vi "采集参数设置 - 副本.vi"() -> ()   [LabVIEW 2020]
panel:
  in  "物理量8下限":sgl format="%#.4g"
  in  "物理量8上限":sgl format="%#.4g"
  in  "物理量7下限":sgl format="%#.4g"
  in  "物理量7上限":sgl format="%#.4g"
  in  "物理量6下限":sgl format="%#.4g"
  in  "物理量6上限":sgl format="%#.4g"
  in  "物理量5下限":sgl format="%#.4g"
  in  "物理量5上限":sgl format="%#.4g"
  in  "物理量4下限":sgl format="%#.4g"
  in  "物理量4上限":sgl format="%#.4g"
  in  "物理量3下限":sgl format="%#.4g"
  in  "物理量3上限":sgl format="%#.4g"
  in  "物理量2下限":sgl format="%#.4g"
  in  "物理量2上限":sgl format="%#.4g"
  in  "物理量1下限":sgl format="%#.4g"
  in  "物理量1上限":sgl format="%#.4g"
  in  "网络服务标尺":u16(ring) items=["计数通量", "电压通量", "电流通量", "棒位", "温度", "P2参数", "硼浓度"]
  in  "端口：":u16=502
  in  "DCS服务器IP地址/主机名：":string="192.168.1.2"
  in  "反应性仪IP地址/主机名：":string="192.168.1.15"
  in  "电压下限8":i32(slide) scale=-10.0..1.0
  in  "电压范围8":i32(slide) scale=1.0..10.0
  in  "电压下限7":i32(slide) scale=-10.0..1.0
  in  "电压范围7":i32(slide) scale=1.0..10.0
  in  "电压下限6":i32(slide) scale=-10.0..1.0
  in  "电压范围6":i32(slide) scale=1.0..10.0
  in  "电压下限5":i32(slide) scale=-10.0..1.0
  in  "电压范围5":i32(slide) scale=1.0..10.0
  in  "电压下限4":i32(slide) scale=-10.0..1.0
  in  "电压范围4":i32(slide) scale=1.0..10.0
  in  "电压下限3":i32(slide) scale=-10.0..1.0
  in  "电压范围3":i32(slide) scale=1.0..10.0
  in  "电压下限2":i32(slide) scale=-10.0..1.0
  in  "电压范围2":i32(slide) scale=1.0..10.0
  in  "电压下限1":i32(slide) scale=-10.0..1.0
  in  "电压范围1":i32(slide) scale=1.0..10.0
  in  "电压标尺8":u16(ring) items=["计数通量LOG", "电压通量", "电流通量LOG", "棒位", "温度", "P2参数", "硼浓度"]
  in  "电压标尺7":u16(ring) items=["计数通量LOG", "电压通量", "电流通量LOG", "棒位", "温度", "P2参数", "硼浓度"]
  in  "电压标尺6":u16(ring) items=["计数通量LOG", "电压通量", "电流通量LOG", "棒位", "温度", "P2参数", "硼浓度"]
  in  "电压标尺5":u16(ring) items=["计数通量LOG", "电压通量", "电流通量LOG", "棒位", "温度", "P2参数", "硼浓度"]
  in  "电压标尺4":u16(ring) items=["计数通量LOG", "电压通量", "电流通量LOG", "棒位", "温度", "P2参数", "硼浓度"]
  in  "电压标尺3":u16(ring) items=["计数通量LOG", "电压通量", "电流通量LOG", "棒位", "温度", "P2参数", "硼浓度"]
  in  "电压标尺2":u16(ring) items=["计数通量LOG", "电压通量", "电流通量LOG", "棒位", "温度", "P2参数", "硼浓度"]
  in  "电压标尺1":u16(ring) items=["计数通量LOG", "电压通量", "电流通量LOG", "棒位", "温度", "P2参数", "硼浓度"]
  in  "电流输入名称2":string
  in  "电流输入名称1":string
  in  "电压输入名称8":string
  in  "电压输入名称7":string
  in  "电压输入名称6":string
  in  "电压输入名称5":string
  in  "电压输入名称4":string
  in  "电压输入名称3":string
  in  "电压输入名称2":string
  in  "电压输入名称1":string
  in  "脉冲输入名称3":string
  in  "脉冲输入名称2":string
  in  "脉冲输入名称1":string
  in  "DCS服务器连接：":bool
  in  "反应性仪连接：":bool
  in  "电流输入2":bool
  in  "电流输入1":bool
  in  "电压输入8":bool
  in  "电压输入7":bool
  in  "电压输入6":bool
  in  "电压输入5":bool
  in  "电压输入4":bool
  in  "恢复":bool caption="Cancel Button"
  out "脉冲3":bool
  out "脉冲2":bool
  in  "电压输入3":bool
  in  "电压输入2":bool
  in  "电压输入1":bool
  out "脉冲1":bool
  in  "脉冲计数通道2":bool
  in  "脉冲计数通道3":bool
  in  "脉冲计数通道1":bool
  in  "取消修改":bool caption="Cancel Button"
  in  "保存修改":bool
  in  "采集时间间隔(s)：":sgl(knob)=0.5 min=0.5 max=2 step=0.5 scale=0.5..2.0 scale format="%#.1f"
  # "仪器硬件通讯设置"
  # "电压输入通道"
  # "电流输入通道"
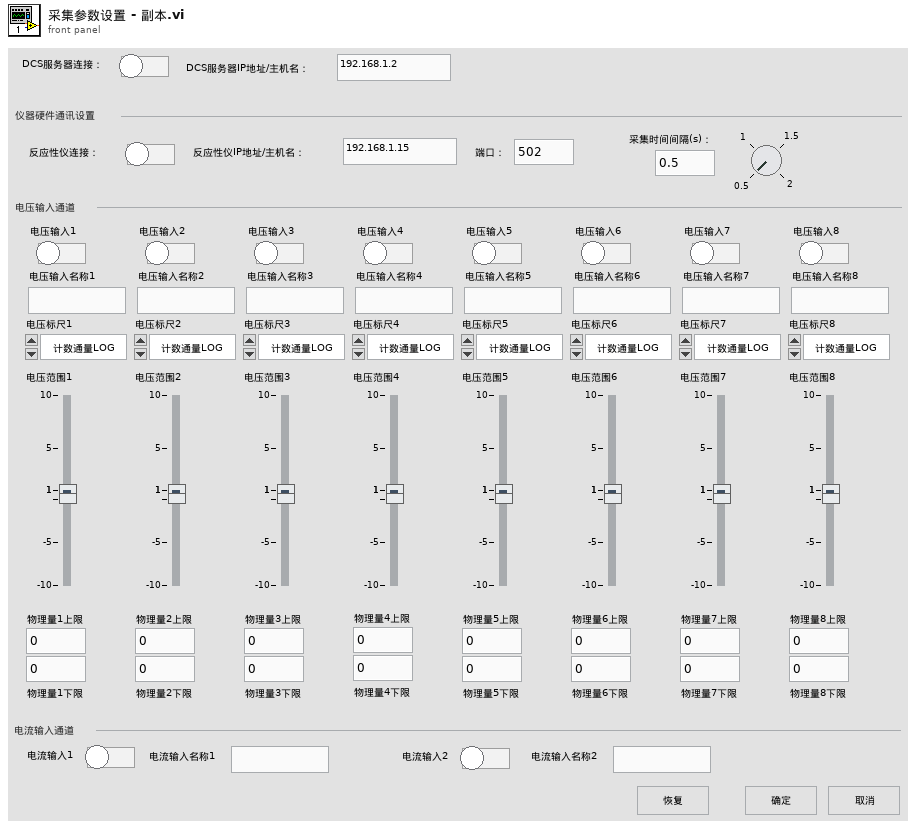
[diagram p1: front panel]
types:
  T1 = enum16{"open", "replace", "create", "open or create", "replace or create", "replace or create with confirmation"}
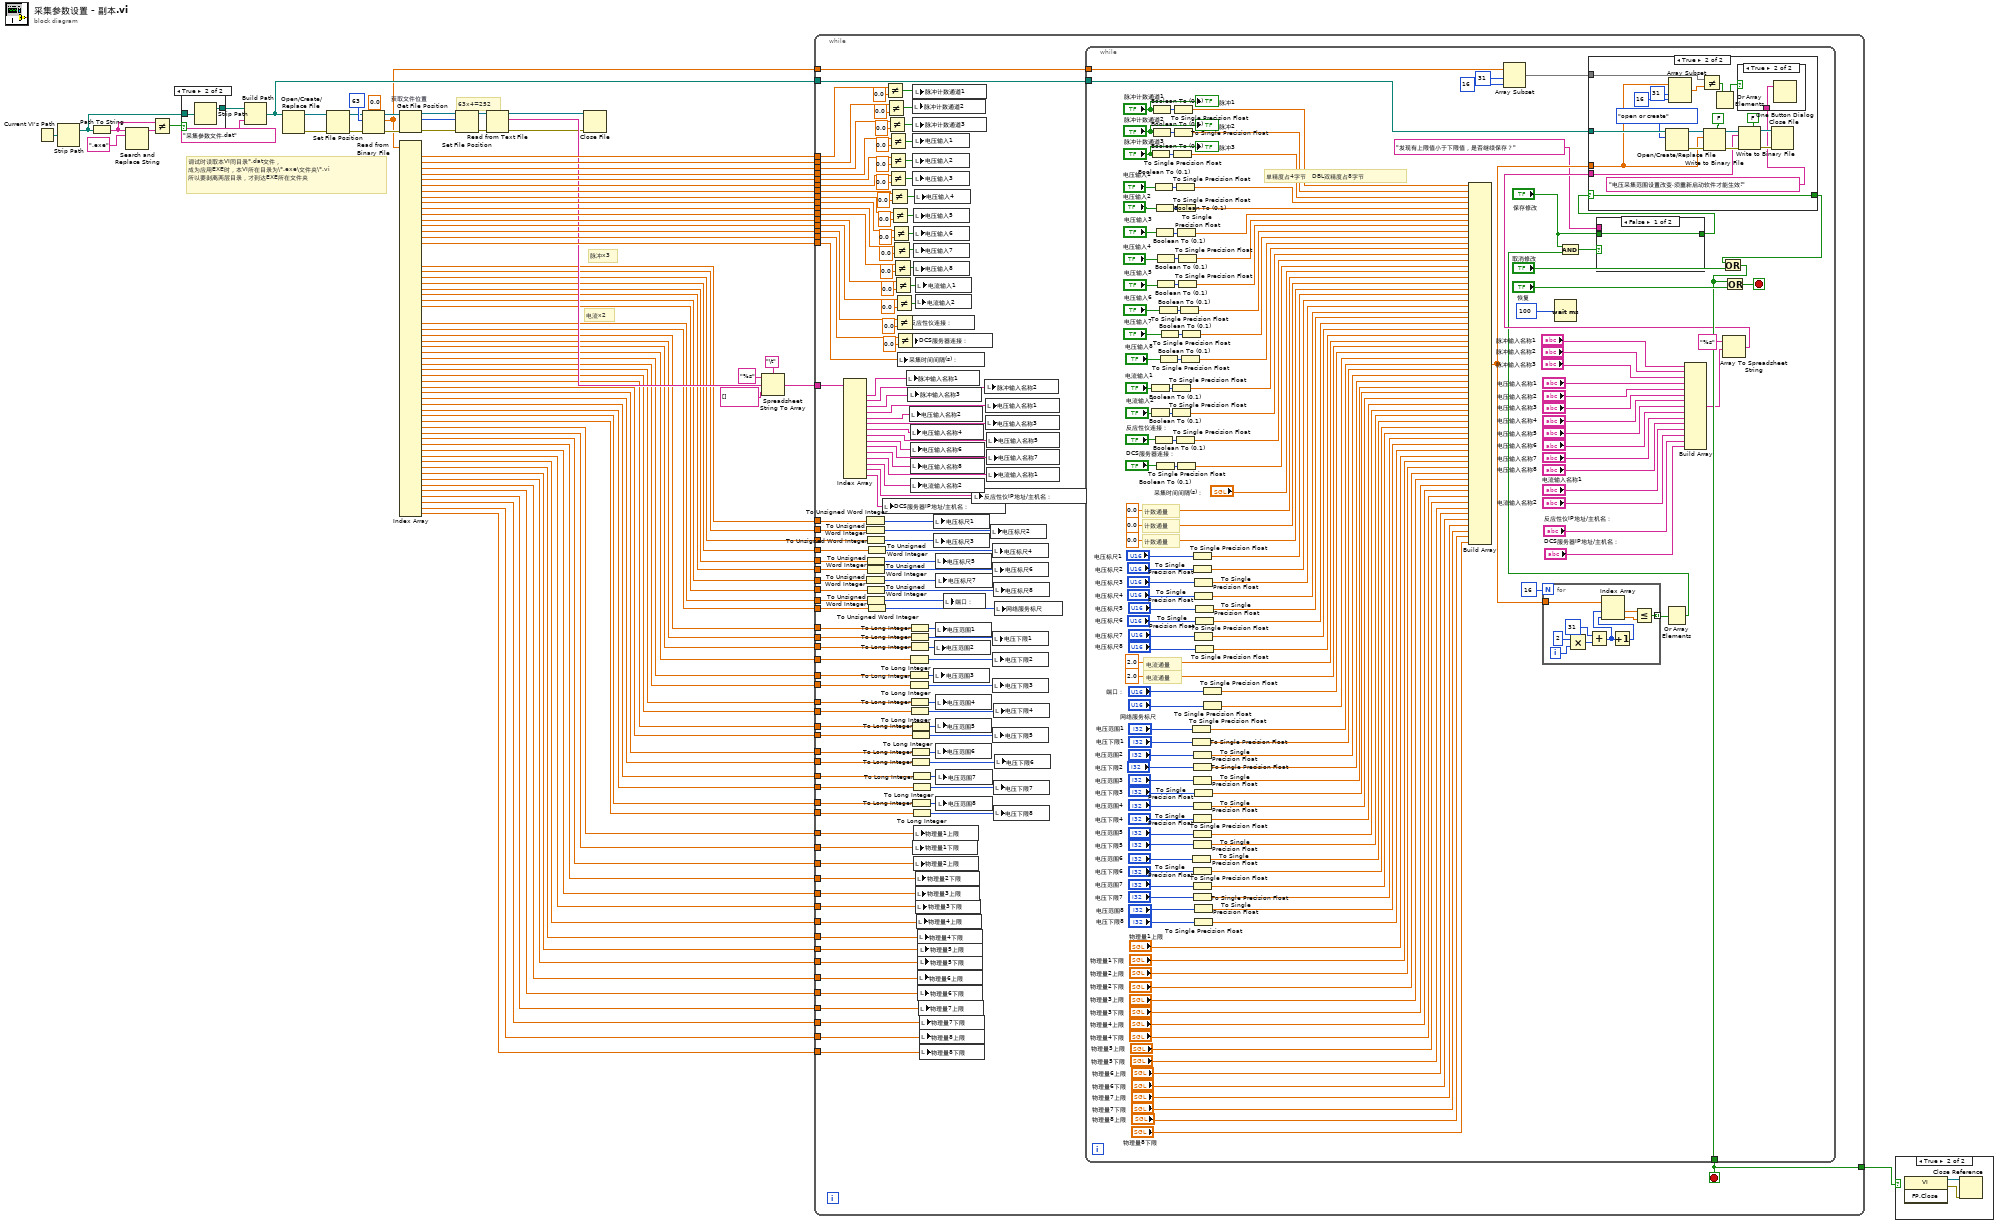
[diagram p0: block diagram]
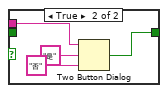
[diagram p4: hidden frame]
diagram:
  # "调试时读取本VI同目录*.dat文件，\n成为应用EXE时，本VI所在目录为\\*.exe\\文件夹\\*.vi\n所以要剥离两层目录，才到达EXE所在文件夹"
  # "63x4=252"
  # "电流x2"
  # "脉冲x3"
  n1 = Current VI's Path() -> (path=w29:path)
  n2 = Strip Path(path=w29) -> (stripped path=w24:path)  [unwired: 1 out]
  n3 = Path To String(path=w24) -> (string=w26:string)
  n4 = Search and Replace String(input string=w26, search string=".exe" ("搜索字符串")) -> (result string=w27:string)  [unwired: 6 in, 3 out]
  n5 = Not Equal?(x=w26, y=w27) -> (x != y?=w25:bool)
  n6 = case shown="True" w25 {
    tunnel: w24 -> [w90 w92]
    tunnel: [w90 w91] -> w23
    frame False {
    }
    frame True {
      n7 = Strip Path(path=w92) -> (stripped path=w91:path)  [unwired: 1 out]
    }
  }
  n8 = Build Path(base path=w23, name or relative path="采集参数文件.dat") -> (appended path=w84:path)
  n9 = Open/Create/Replace File(file path (use dialog)=w84) -> (refnum out=w67:refnum<file>, error out=w66:errorcluster)  [unwired: 5 in, 1 out]
  n10 = Set File Position(refnum=w67, error in=w66) -> (refnum out=w65:refnum<file>, error out=w64:errorcluster)  [unwired: 2 in]
  n11 = Read from Binary File(5:sgl 0.0 ("byte stream type"), 8:w64, 10:63 ("count"), 11:w65) -> (0:w82:errorcluster, 2:w4:sgl[], 3:w83:refnum<file>)  [unwired: 2 in, 1 out]
  n12 = Get File Position "获取文件位置"(4:w82, 7:w83) -> (0:w86:errorcluster, 2:w52:i64, 3:w87:refnum<file>)
  n13 = Index Array(array=w4) -> (element #1=w81:sgl, element #2=w80:sgl, element #3=w79:sgl, element #4=w78:sgl, element #5=w77:sgl, element #6=w76:sgl, element #7=w75:sgl, element #8=w74:sgl, element #9=w73:sgl, element #10=w72:sgl, element #11=w71:sgl, element #12=w70:sgl, element #13=w69:sgl, element #14=w68:sgl, element #15=w63:sgl, element #16=w62:sgl, element #20=w51:sgl, element #21=w50:sgl, element #22=w49:sgl, element #23=w48:sgl, element #24=w47:sgl, element #25=w46:sgl, element #26=w45:sgl, element #27=w44:sgl, element #30=w2:sgl, element #31=w3:sgl, element #32=w43:sgl, element #33=w42:sgl, element #34=w41:sgl, element #35=w40:sgl, element #36=w21:sgl, element #37=w22:sgl, element #38=w39:sgl, element #39=w38:sgl, element #40=w37:sgl, element #41=w36:sgl, element #42=w35:sgl, element #43=w34:sgl, element #44=w33:sgl, element #45=w32:sgl, element #46=w31:sgl, element #47=w30:sgl, element #48=w20:sgl, element #49=w19:sgl, element #50=w18:sgl, element #51=w17:sgl, element #52=w16:sgl, element #53=w15:sgl, element #54=w14:sgl, element #55=w13:sgl, element #56=w12:sgl, element #57=w11:sgl, element #58=w10:sgl, element #59=w9:sgl, element #60=w8:sgl, element #61=w7:sgl, element #62=w6:sgl, element #63=w5:sgl)  [unwired: 63 in, 5 out]
  n14 = Set File Position(offset (in bytes) (0)=w52, refnum=w87, error in=w86) -> (refnum out=w59:refnum<file>, error out=w58:errorcluster)  [unwired: 1 in]
  n15 = Read from Text File(file (use dialog)=w59, error in=w58) -> (refnum out=w54:refnum<file>, text=w57:string, error out=w55:errorcluster)  [unwired: 1 in, 2 out]
  n16 = Close File(refnum=w54, error in=w55) -> ()  [unwired: 2 out]
  n17 = Spreadsheet String To Array(delimiter (Tab)="\t", format string="%s", spreadsheet string=w57, array type (2D Dbl)=string[] [] ("添加的数组")) -> (array=w53:string[])
  n18 = while {
    tunnel: w81 -> [w224]
    tunnel: w80 -> [w218]
    tunnel: w79 -> [w217]
    tunnel: w78 -> [w216]
    tunnel: w77 -> [w210]
    tunnel: w76 -> [w208]
    tunnel: w75 -> [w196]
    tunnel: w74 -> [w195]
    tunnel: w73 -> [w194]
    tunnel: w72 -> [w193]
    tunnel: w71 -> [w192]
    tunnel: w70 -> [w183]
    tunnel: w84 -> [w225]
    tunnel: w69 -> [w182]
    tunnel: w68 -> [w181]
    tunnel: w63 -> [w180]
    tunnel: w62 -> [w179]
    tunnel: w53 -> [w178]
    tunnel: w51 -> [w156]
    tunnel: w50 -> [w155]
    tunnel: w49 -> [w154]
    tunnel: w48 -> [w153]
    tunnel: w47 -> [w152]
    tunnel: w46 -> [w151]
    tunnel: w45 -> [w150]
    tunnel: w44 -> [w149]
    tunnel: w2 -> [w114]
    tunnel: w3 -> [w113]
    tunnel: w41 -> [w132]
    tunnel: w40 -> [w131]
    tunnel: w21 -> [w130]
    tunnel: w22 -> [w129]
    tunnel: w39 -> [w128]
    tunnel: w38 -> [w127]
    tunnel: w37 -> [w126]
    tunnel: w36 -> [w125]
    tunnel: w35 -> [w124]
    tunnel: w34 -> [w123]
    tunnel: w33 -> [w122]
    tunnel: w32 -> [w121]
    tunnel: w31 -> [w120]
    tunnel: w30 -> [w119]
    tunnel: w43 -> [w112]
    tunnel: w42 -> [w111]
    tunnel: w20 -> [w110]
    tunnel: w19 -> [w109]
    tunnel: w18 -> [w108]
    tunnel: w17 -> [w107]
    tunnel: w16 -> [w106]
    tunnel: w15 -> [w105]
    tunnel: w14 -> [w104]
    tunnel: w13 -> [w103]
    tunnel: w12 -> [w102]
    tunnel: w11 -> [w101]
    tunnel: w10 -> [w100]
    tunnel: w9 -> [w99]
    tunnel: w8 -> [w98]
    tunnel: w7 -> [w97]
    tunnel: w6 -> [w96]
    tunnel: w5 -> [w95]
    tunnel: w4 -> [w94]
    tunnel: [w93] -> w1
    stop <- w93 stop-if-true
    n19 = Index Array(array=w178) -> (element #1=w177:string, element #2=w176:string, element #3=w175:string, element #4=w174:string, element #5=w173:string, element #6=w172:string, element #7=w171:string, element #8=w170:string, element #9=w169:string, element #10=w168:string, element #11=w167:string, element #12=w165:string, element #13=w166:string, element #14=w118:string, element #15=w117:string)  [unwired: 15 in]
    n20 = To Unsigned Word Integer(number=w156) -> (unsigned 16bit integer=w164:u16)
    n21 = To Unsigned Word Integer(number=w155) -> (unsigned 16bit integer=w162:u16)
    n22 = To Unsigned Word Integer(number=w150) -> (unsigned 16bit integer=w158:u16)
    n23 = To Unsigned Word Integer(number=w154) -> (unsigned 16bit integer=w163:u16)
    n24 = To Unsigned Word Integer(number=w152) -> (unsigned 16bit integer=w160:u16)
    n25 = To Unsigned Word Integer(number=w151) -> (unsigned 16bit integer=w159:u16)
    n26 = To Unsigned Word Integer(number=w149) -> (unsigned 16bit integer=w157:u16)
    n27 = To Unsigned Word Integer(number=w114) -> (unsigned 16bit integer=w116:u16)
    n28 = To Unsigned Word Integer(number=w153) -> (unsigned 16bit integer=w161:u16)
    n29 = To Unsigned Word Integer(number=w113) -> (unsigned 16bit integer=w115:u16)
    n30 = local write "DCS服务器IP地址/主机名："(w117) -> ()
    n31 = Not Equal?(x=w224, y=sgl 0.0) -> (x != y?=w222:bool)
    n32 = Not Equal?(x=w218, y=sgl 0.0) -> (x != y?=w215:bool)
    n33 = Not Equal?(x=w217, y=sgl 0.0) -> (x != y?=w214:bool)
    n34 = Not Equal?(x=w216, y=sgl 0.0) -> (x != y?=w213:bool)
    n35 = Not Equal?(x=w210, y=sgl 0.0) -> (x != y?=w211:bool)
    n36 = Not Equal?(x=w208, y=sgl 0.0) -> (x != y?=w207:bool)
    n37 = Not Equal?(x=w196, y=sgl 0.0) -> (x != y?=w201:bool)
    n38 = Not Equal?(x=w195, y=sgl 0.0) -> (x != y?=w200:bool)
    n39 = Not Equal?(x=w194, y=sgl 0.0) -> (x != y?=w199:bool)
    n40 = Not Equal?(x=w193, y=sgl 0.0) -> (x != y?=w198:bool)
    n41 = Not Equal?(x=w192, y=sgl 0.0) -> (x != y?=w197:bool)
    n42 = Not Equal?(x=w183, y=sgl 0.0) -> (x != y?=w185:bool)
    n43 = Not Equal?(x=w182, y=sgl 0.0) -> (x != y?=w184:bool)
    n44 = Not Equal?(x=w181, y=sgl 0.0) -> (x != y?=w189:bool)
    n45 = Not Equal?(x=w180, y=sgl 0.0) -> (x != y?=w188:bool)
    n46 = local write "采集时间间隔(s)："(w179) -> ()
    n47 = local write "反应性仪连接："(w189) -> ()
    n48 = local write "脉冲输入名称1"(w177) -> ()
    n49 = local write "DCS服务器连接："(w188) -> ()
    n50 = local write "脉冲输入名称3"(w175) -> ()
    n51 = To Long Integer(number=w131) -> (32bit integer=w139:i32)
    n52 = To Long Integer(number=w130) -> (32bit integer=w146:i32)
    n53 = To Long Integer(number=w129) -> (32bit integer=w138:i32)
    n54 = To Long Integer(number=w112) -> (32bit integer=w148:i32)
    n55 = To Long Integer(number=w111) -> (32bit integer=w140:i32)
    n56 = To Long Integer(number=w132) -> (32bit integer=w147:i32)
    n57 = To Long Integer(number=w128) -> (32bit integer=w145:i32)
    n58 = To Long Integer(number=w127) -> (32bit integer=w137:i32)
    n59 = local write "电压输入名称2"(w173) -> ()
    n60 = To Long Integer(number=w126) -> (32bit integer=w144:i32)
    n61 = To Long Integer(number=w125) -> (32bit integer=w136:i32)
    n62 = To Long Integer(number=w124) -> (32bit integer=w143:i32)
    n63 = To Long Integer(number=w123) -> (32bit integer=w135:i32)
    n64 = local write "电压输入名称4"(w171) -> ()
    n65 = To Long Integer(number=w120) -> (32bit integer=w141:i32)
    n66 = local write "电压输入名称6"(w169) -> ()
    n67 = local write "电压输入名称8"(w167) -> ()
    n68 = local write "电流输入名称2"(w166) -> ()
    n69 = To Long Integer(number=w122) -> (32bit integer=w142:i32)
    n70 = To Long Integer(number=w121) -> (32bit integer=w134:i32)
    n71 = To Long Integer(number=w119) -> (32bit integer=w133:i32)
    n72 = local write "脉冲计数通道2"(w215) -> ()
    n73 = local write "脉冲计数通道1"(w222) -> ()
    n74 = local write "脉冲计数通道3"(w214) -> ()
    n75 = local write "电压输入1"(w213) -> ()
    n76 = local write "电压输入2"(w211) -> ()
    n77 = local write "电压输入3"(w207) -> ()
    n78 = local write "物理量1下限"(w109) -> ()
    n79 = local write "电压输入5"(w200) -> ()
    n80 = local write "电压输入6"(w199) -> ()
    n81 = local write "电压输入7"(w198) -> ()
    n82 = local write "电压输入8"(w197) -> ()
    n83 = local write "物理量1上限"(w110) -> ()
    n84 = local write "物理量2上限"(w108) -> ()
    n85 = local write "电压输入4"(w201) -> ()
    n86 = local write "电流输入2"(w184) -> ()
    n87 = local write "物理量2下限"(w107) -> ()
    n88 = local write "物理量3上限"(w106) -> ()
    n89 = local write "电流输入1"(w185) -> ()
    n90 = local write "物理量3下限"(w105) -> ()
    n91 = local write "物理量4上限"(w104) -> ()
    n92 = local write "物理量4下限"(w103) -> ()
    n93 = local write "物理量6上限"(w100) -> ()
    n94 = local write "物理量5上限"(w102) -> ()
    n95 = local write "物理量5下限"(w101) -> ()
    n96 = local write "物理量6下限"(w99) -> ()
    n97 = local write "物理量7上限"(w98) -> ()
    n98 = local write "物理量7下限"(w97) -> ()
    n99 = local write "物理量8上限"(w96) -> ()
    n100 = local write "物理量8下限"(w95) -> ()
    n101 = local write "电压标尺1"(w164) -> ()
    n102 = local write "电压标尺3"(w163) -> ()
    n103 = local write "电压范围3"(w146) -> ()
    n104 = local write "电压范围2"(w147) -> ()
    n105 = local write "电压标尺5"(w160) -> ()
    n106 = local write "电压范围1"(w148) -> ()
    n107 = local write "电压范围4"(w145) -> ()
    n108 = local write "电压范围5"(w144) -> ()
    n109 = local write "电压范围6"(w143) -> ()
    n110 = local write "电压标尺7"(w158) -> ()
    n111 = local write "电压范围7"(w142) -> ()
    n112 = local write "电压范围8"(w141) -> ()
    n113 = local write "端口："(w116) -> ()
    n114 = local write "反应性仪IP地址/主机名："(w118) -> ()
    n115 = local write "脉冲输入名称2"(w176) -> ()
    n116 = local write "电压输入名称1"(w174) -> ()
    n117 = local write "电压输入名称3"(w172) -> ()
    n118 = local write "电压输入名称5"(w170) -> ()
    n119 = local write "电压输入名称7"(w168) -> ()
    n120 = local write "电流输入名称1"(w165) -> ()
    n121 = local write "电压标尺2"(w162) -> ()
    n122 = local write "电压标尺4"(w161) -> ()
    n123 = local write "电压下限1"(w140) -> ()
    n124 = local write "电压标尺6"(w159) -> ()
    n125 = local write "电压下限2"(w139) -> ()
    n126 = local write "电压下限3"(w138) -> ()
    n127 = local write "电压下限5"(w136) -> ()
    n128 = local write "电压标尺8"(w157) -> ()
    n129 = local write "电压下限4"(w137) -> ()
    n130 = local write "电压下限7"(w134) -> ()
    n131 = local write "电压下限8"(w133) -> ()
    n132 = local write "网络服务标尺"(w115) -> ()
    n133 = local write "电压下限6"(w135) -> ()
    n134 = while {
      tunnel: w225 -> [w381]
      tunnel: [w357] -> w93
      tunnel: w94 -> [w232]
      stop <- w358 stop-if-true
      # "电流通量"
      # "电流通量"
      # "计数通量"
      # "计数通量"
      # "计数通量"
      # "单精度占4字节   DBL双精度占8字节"
      n135 = Boolean To (0,1)(Boolean="电流输入1") -> (0, 1=w343:i16)
      n136 = Boolean To (0,1)(Boolean="电流输入2") -> (0, 1=w342:i16)
      n137 = Boolean To (0,1)(Boolean="脉冲计数通道3") -> (0, 1=w378:i16)
      n138 = Boolean To (0,1)(Boolean="脉冲计数通道1") -> (0, 1=w380:i16)
      n139 = Boolean To (0,1)(Boolean="脉冲计数通道2") -> (0, 1=w379:i16)
      n140 = Boolean To (0,1)(Boolean="电压输入1") -> (0, 1=w377:i16)
      n141 = Boolean To (0,1)(Boolean="反应性仪连接：") -> (0, 1=w335:i16)
      n142 = Boolean To (0,1)(Boolean="电压输入2") -> (0, 1=w372:i16)
      n143 = Boolean To (0,1)(Boolean="电压输入3") -> (0, 1=w371:i16)
      n144 = Boolean To (0,1)(Boolean="DCS服务器连接：") -> (0, 1=w334:i16)
      n145 = Boolean To (0,1)(Boolean="电压输入4") -> (0, 1=w347:i16)
      n146 = Boolean To (0,1)(Boolean="电压输入5") -> (0, 1=w348:i16)
      n147 = Boolean To (0,1)(Boolean="电压输入6") -> (0, 1=w349:i16)
      n148 = Boolean To (0,1)(Boolean="电压输入8") -> (0, 1=w351:i16)
      n149 = Boolean To (0,1)(Boolean="电压输入7") -> (0, 1=w350:i16)
      n150 = To Single Precision Float(number=w343) -> (single precision float=w339:sgl)
      n151 = To Single Precision Float(number=w342) -> (single precision float=w338:sgl)
      n152 = To Single Precision Float(number=w378) -> (single precision float=w374:sgl)
      n153 = To Single Precision Float(number=w380) -> (single precision float=w376:sgl)
      n154 = To Single Precision Float(number=w379) -> (single precision float=w375:sgl)
      n155 = To Single Precision Float(number=w377) -> (single precision float=w373:sgl)
      n156 = To Single Precision Float(number=w335) -> (single precision float=w331:sgl)
      n157 = To Single Precision Float(number=w372) -> (single precision float=w370:sgl)
      n158 = To Single Precision Float(number=w371) -> (single precision float=w369:sgl)
      n159 = To Single Precision Float(number=w334) -> (single precision float=w330:sgl)
      n160 = To Single Precision Float(number=w347) -> (single precision float=w346:sgl)
      n161 = To Single Precision Float(number=w348) -> (single precision float=w336:sgl)
      n162 = To Single Precision Float(number=w349) -> (single precision float=w345:sgl)
      n163 = To Single Precision Float(number=w351) -> (single precision float=w337:sgl)
      n164 = To Single Precision Float(number=w350) -> (single precision float=w344:sgl)
      n165 = To Single Precision Float(number="电压范围1") -> (single precision float=w269:sgl)
      n166 = To Single Precision Float(number="电压下限1") -> (single precision float=w268:sgl)
      n167 = To Single Precision Float(number="电压范围6") -> (single precision float=w259:sgl)
      n168 = To Single Precision Float(number="电压标尺1") -> (single precision float=w283:sgl)
      n169 = To Single Precision Float(number="电压标尺2") -> (single precision float=w282:sgl)
      n170 = To Single Precision Float(number="电压范围2") -> (single precision float=w267:sgl)
      n171 = To Single Precision Float(number="电压下限2") -> (single precision float=w266:sgl)
      n172 = To Single Precision Float(number="电压范围3") -> (single precision float=w265:sgl)
      n173 = To Single Precision Float(number="电压范围4") -> (single precision float=w263:sgl)
      n174 = To Single Precision Float(number="电压下限4") -> (single precision float=w262:sgl)
      n175 = To Single Precision Float(number="电压范围5") -> (single precision float=w261:sgl)
      n176 = To Single Precision Float(number="电压下限5") -> (single precision float=w260:sgl)
      n177 = To Single Precision Float(number="电压下限6") -> (single precision float=w258:sgl)
      n178 = To Single Precision Float(number="电压范围7") -> (single precision float=w257:sgl)
      n179 = To Single Precision Float(number="电压下限7") -> (single precision float=w256:sgl)
      n180 = To Single Precision Float(number="电压标尺3") -> (single precision float=w281:sgl)
      n181 = To Single Precision Float(number="电压标尺4") -> (single precision float=w280:sgl)
      n182 = To Single Precision Float(number="电压标尺7") -> (single precision float=w277:sgl)
      n183 = To Single Precision Float(number="电压下限3") -> (single precision float=w264:sgl)
      n184 = To Single Precision Float(number="电压范围8") -> (single precision float=w255:sgl)
      n185 = To Single Precision Float(number="电压下限8") -> (single precision float=w254:sgl)
      n186 = To Single Precision Float(number="电压标尺5") -> (single precision float=w279:sgl)
      n187 = To Single Precision Float(number="电压标尺6") -> (single precision float=w278:sgl)
      n188 = To Single Precision Float(number="电压标尺8") -> (single precision float=w276:sgl)
      n189 = To Single Precision Float(number="端口：") -> (single precision float=w271:sgl)
      n190 = To Single Precision Float(number="网络服务标尺") -> (single precision float=w270:sgl)
      n191 = Build Array(w376, w375, w374, w373, w370, w369, w346, w336, w345, w344, w337, w339, w338, w331, w330, "采集时间间隔(s)：", sgl 0.0 ("单精度浮点"), sgl 0.0 ("单精度浮点"), sgl 0.0 ("单精度浮点"), w283, w282, w281, w280, w279, w278, w277, w276, sgl 2.0 ("单精度浮点"), sgl 2.0 ("单精度浮点"), w271, w270, w269, w268, w267, w266, w265, w264, w263, w262, w261, w260, w259, w258, w257, w256, w255, w254, "物理量1上限", "物理量1下限", "物理量2上限", "物理量2下限", "物理量3上限", "物理量3下限", "物理量4上限", "物理量4下限", "物理量5上限", "物理量5下限", "物理量6上限", "物理量6下限", "物理量7上限", "物理量7下限", "物理量8上限", "物理量8下限") -> (w234:sgl[])
      n192 = Array Subset(array=w232, index=31 ("索引"), length=16 ("长度")) -> (w235:sgl[])
      n193 = for {
        N: 16 -> [_]
        tunnel: w234 -> [w392]
        tunnel: [w387] -> w231 mode=indexing
        i -> [w396]
        n194 = Multiply(x=2, y=w396) -> (x*y=w394:i32)
        n195 = Add(x=31, y=w394) -> (x+y=w389:i32)
        n196 = Increment(x=w389) -> (x+1=w388:i32)
        n197 = Index Array(array=w392, index #1=w389, index #2=w388) -> (element #1=w391:sgl, element #2=w390:sgl)
        n198 = Less Or Equal?(x=w391, y=w390) -> (x <= y?=w387:bool)
      }
      n199 = Wait (ms)(milliseconds to wait=u32 100 ("等待时间（毫秒）")) -> ()  [unwired: 1 out]
      n200 = Or Array Elements(Boolean array=w231) -> (logical OR=w228:bool)
      n201 = And(x="保存修改", y=w228) -> (x .and. y?=w227:bool)
      n202 = case shown="False" w227 {
        tunnel: [w382 w383] -> w230
        tunnel: "发现有上限值小于下限值，是否继续保存？" ("消息") -> [_ w384]
        tunnel: "保存修改" -> [w382 _]
        frame False {
        }
        frame True {
          n203 = Two Button Dialog(message=w384, 1:"否" ("按钮名称（“确定”）"), 2:"是" ("T按钮名称（“确定”）")) -> (T button?=w383:bool)
        }
      }
      n204 = Build Array("脉冲输入名称1", "脉冲输入名称2", "脉冲输入名称3", "电压输入名称1", "电压输入名称2", "电压输入名称3", "电压输入名称4", "电压输入名称5", "电压输入名称6", "电压输入名称7", "电压输入名称8", "电流输入名称1", "电流输入名称2", "反应性仪IP地址/主机名：", "DCS服务器IP地址/主机名：") -> (w313:string[])
      n205 = Array To Spreadsheet String(array=w313, 3:"%s" ("format string")) -> (spreadsheet string=w327:string)  [unwired: 1 in]
      n206 = case shown="True" w230 {
        selector: w230 -> [w397 w412]
        tunnel: w381 -> [_ w417]
        tunnel: w234 -> [_ w403]
        tunnel: [w397 w412] -> w362
        tunnel: w327 -> [_ w406]
        tunnel: w235 -> [_ w402]
        frame False {
        }
        frame True {
          n207 = Open/Create/Replace File(file path (use dialog)=w417, operation (0:open)=T1."open or create" ("操作(0:open)")) -> (refnum out=w416:refnum<file>, error out=w415:errorcluster)  [unwired: 4 in, 1 out]
          n208 = Array Subset(array=w403, index=31 ("索引"), length=16 ("长度")) -> (w401:sgl[])
          n209 = Not Equal?(x=w402, y=w401) -> (x != y?=w400:bool[])
          n210 = Write to Binary File(file (use dialog)=w416, data=w403, error in=w415, 5:FALSE ("预置数组或字符串大小？(T)")) -> (refnum out=w409:refnum<file>, error out=w411:errorcluster)  [unwired: 2 in, 1 out]
          n211 = Or Array Elements(Boolean array=w400) -> (logical OR=w399:bool)
          n212 = case shown="True" w399 {
            tunnel: "电压采集范围设置改变,须重新启动软件才能生效!" ("spreadsheet string") -> [_ w418]
            frame False {
            }
            frame True {
              n213 = One Button Dialog(message=w418) -> ()  [unwired: 1 in, 1 out]
            }
          }
          n214 = Write to Binary File(file (use dialog)=w409, data=w406, error in=w411, 5:FALSE ("预置数组或字符串大小？(T)")) -> (refnum out=w408:refnum<file>, error out=w410:errorcluster)  [unwired: 2 in, 1 out]
          n215 = Close File(refnum=w408, error in=w410) -> ()  [unwired: 2 out]
        }
      }
      n216 = Or(x=w362, y="取消修改") -> (x .or. y?=w357:bool)
      n217 = Or(x=w357, y="恢复") -> (x .or. y?=w358:bool)
      "脉冲1" <- "脉冲计数通道1"
      "脉冲2" <- "脉冲计数通道2"
      "脉冲3" <- "脉冲计数通道3"
    }
  }
  n218 = case shown="True" w1 {
    frame False {
    }
    frame True {
      n219 = invoke class="VI" method="FP.Close"() -> (reference out=w419:refnum<vi>, error out=w420:errorcluster)  [unwired: 3 in, 1 out]
      n220 = Close Reference(reference=w419, error in (no error)=w420) -> ()  [unwired: 1 out]
    }
  }
